vi "SENS_SEGM_DEL_ALL.vi"(0 "VISA IN":refnum<visa-resource-name>, 5 "error in":errorcluster, 7 "Channel":i32) -> (14 "VISA Out":refnum<visa-resource-name>, 19 "error out":errorcluster)   [LabVIEW 2018, in "PNA-X.lvlib"]
doc: "SENSe<cnum>:SEGMent:DELete:ALL \n(Write-only) Deletes all sweep segments. When this command is executed, Sweep Mode \n(SENS:SWE:MODE) is automatically set to Linear because there are no segments to sweep. \nParameters \n<cnum> Any existing channel number. If unspecified, value is set to 1 \nExamples SENS:SEGM:DEL:ALL \nsense2:segment:delete:all \nQuery Syntax Not applicable \nDefault Not Applicable"
uses:
  PNA-X.lvlib
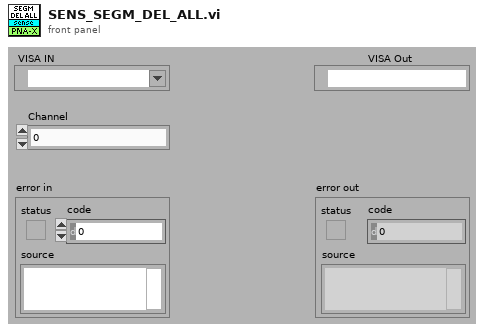
[diagram p1: front panel]
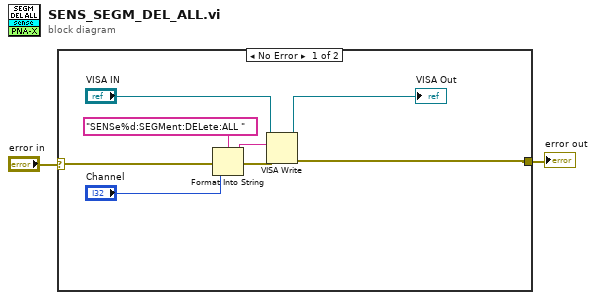
[diagram p0: block diagram]
diagram:
  n1 = case shown="No Error" "error in" {
    selector: "error in" -> [w10 w11]
    tunnel: [w5 w11] -> w1
    frame No Error {
      n2 = Format Into String(format string="SENSe%d:SEGMent:DELete:ALL " ("Cmdline"), error in=w10, "Channel") -> (resulting string=w8:string, error out=w9:errorcluster)  [unwired: 1 in]
      n3 = VISA Write(VISA resource name="VISA IN", write buffer=w8, error in (no error)=w9) -> (VISA resource name out=→"VISA Out":refnum<visa-resource-name>, error out=w5:errorcluster)  [unwired: 1 out]
    }
    frame Error {
    }
  }
  "error out" <- w1
